vi "laba 9.vi"() -> ()   [LabVIEW 2010]
doc: "Use this template to build a producer/consumer design pattern with events to produce queue items. Use this design pattern instead of the User Interface Event Handler pattern for user interfaces when you want to execute code asynchronously in response to an event without slowing the user interface responsiveness."
uses:
  laba_9_typedef.ctl
panel:
  in  "Start":bool
  out "string":string
  in  "Stop":bool
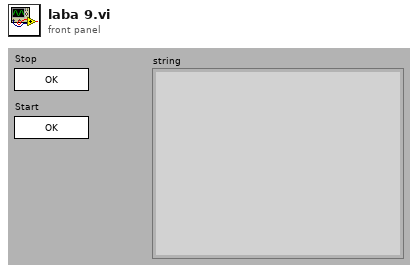
[diagram p1: front panel]
types:
  T1 = typedef "laba_9_typedef.ctl" = enum16{"Initialize", "Read multi", "String view", "Stop"}
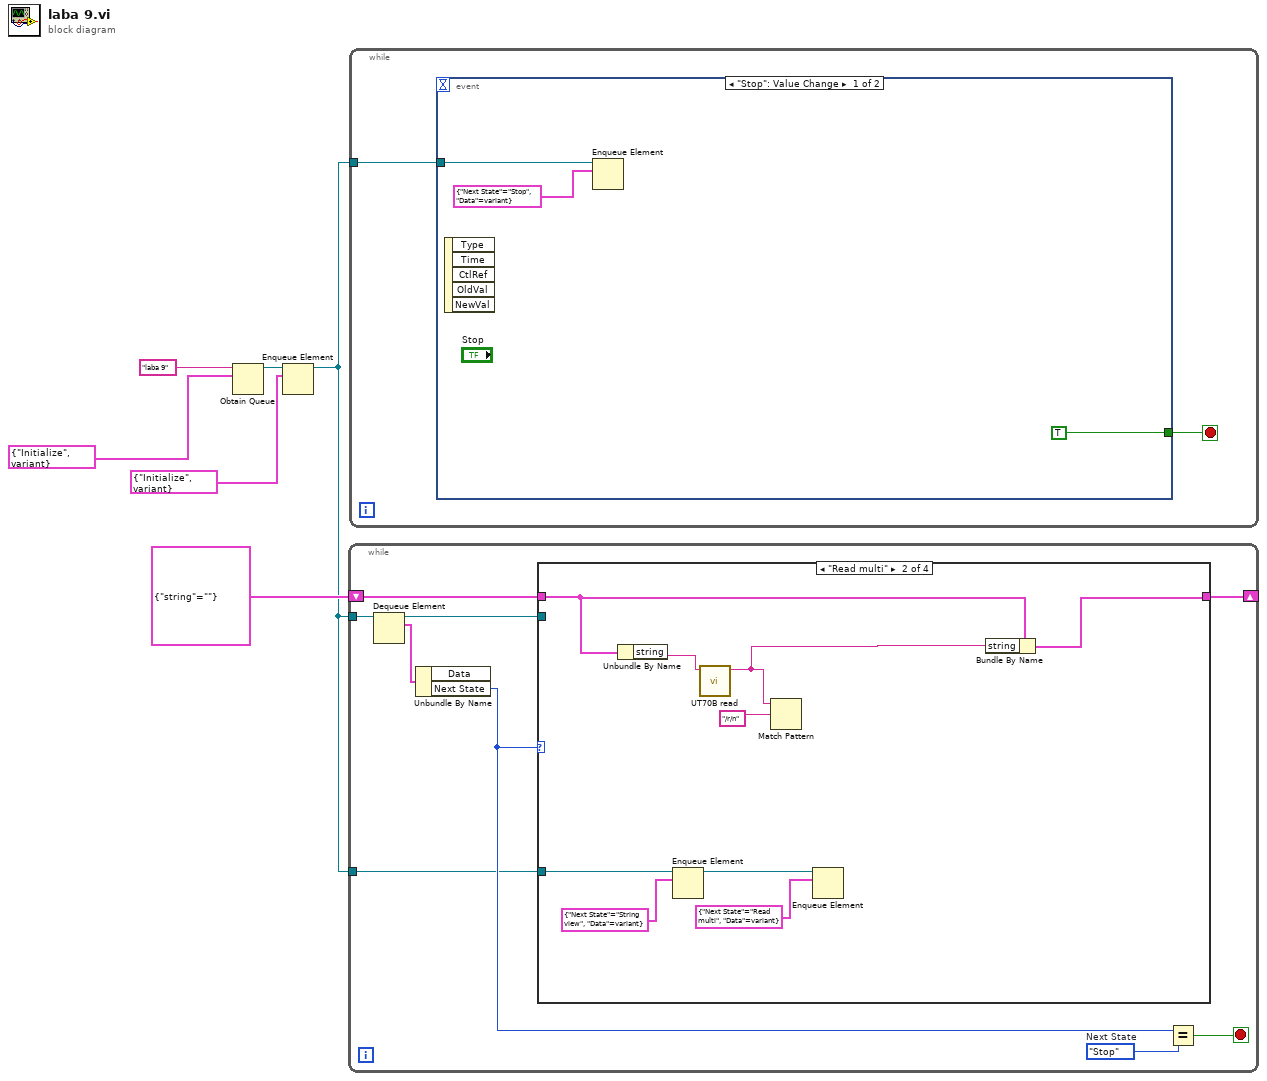
[diagram p0: block diagram]
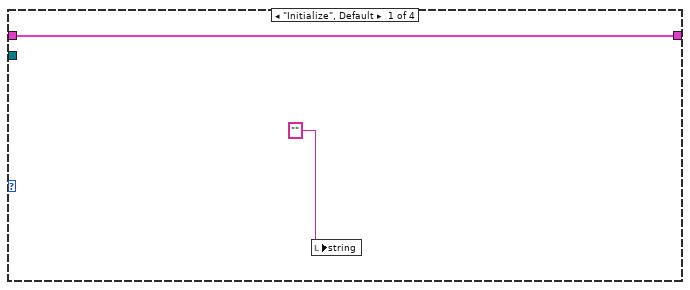
[diagram p2: hidden frame]
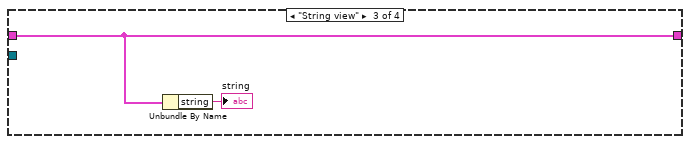
[diagram p3: hidden frame]
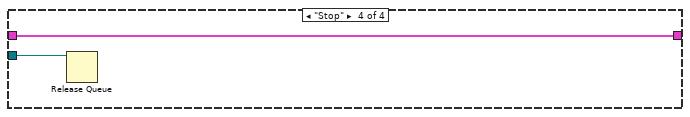
[diagram p4: hidden frame]
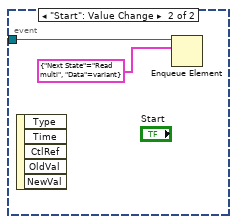
[diagram p5: hidden frame]
diagram:
  n1 = Obtain Queue(name (unnamed)="laba 9", element data type=cluster{"Next State":T1, "Data":variant} {"Next State"=enum."Initialize", "Data"=variant}) -> (queue out=w6:refnum<queue>)  [unwired: 3 in, 2 out]
  n2 = Enqueue Element(queue=w6, element=cluster{"Next State":T1, "Data":variant} {"Next State"=enum."Initialize", "Data"=variant}) -> (queue out=w1:refnum<queue>)  [unwired: 2 in, 2 out]
  n3 = while {
    tunnel: w1 -> [w15]
    shift-right: [w8] -> _
    shift-left: cluster{"string":string} {"string"=""} -> [w9]
    tunnel: w1 -> [w7]
    stop <- w13 stop-if-true
    w12 = laba_9_typedef."Stop"  # Next State
    n4 = Dequeue Element(queue=w15) -> (queue out=w10:refnum<queue>, element=w14:cluster{"Next State":T1, "Data":variant})  [unwired: 2 in, 2 out]
    n5 = Unbundle By Name(w14) -> ("Next State"=w11:T1)  [unwired: 1 out]
    n6 = case shown="\"Read multi\"" w11 {
      tunnel: w10 -> [_ _ _ w30]
      tunnel: w9 -> [w17 w25 w28 w29]
      tunnel: [w17 w24 w28 w29] -> w8
      tunnel: w7 -> [_ w23 _ _]
      frame "Initialize", Default {
        n7 = local write "string"("" ("string")) -> ()
      }
      frame "Read multi" {
        n8 = Unbundle By Name(w25) -> ("string"=w26:string)
        n9 = Enqueue Element(queue=w23, element=cluster{"Next State":T1, "Data":variant} {"Next State"=enum."String view", "Data"=variant}) -> (queue out=w21:refnum<queue>)  [unwired: 2 in, 2 out]
        n10 = call "UT70B read.vi"("string in"=w26) -> ("string out"=w19:string)  [unwired: 10 in]
        n11 = Match Pattern(string=w19, regular expression="/r/n") -> ()  [unwired: 1 in, 4 out]
        n12 = Enqueue Element(queue=w21, element=cluster{"Next State":T1, "Data":variant} {"Next State"=enum."Read multi", "Data"=variant}) -> ()  [unwired: 2 in, 3 out]
        n13 = Bundle By Name(cluster=w25, "string"=w19) -> (w24:cluster{"string":string})
      }
      frame "String view" {
        n14 = Unbundle By Name(w28) -> ("string"=→"string":string)
      }
      frame "Stop" {
        n15 = Release Queue(queue=w30) -> ()  [unwired: 2 in, 3 out]
      }
    }
    n16 = Equal?(x=w11, y=w12) -> (x = y?=w13:bool)
  }
  n17 = while {
    tunnel: w1 -> [w32]
    stop <- w31 stop-if-true
    n18 = event shown="[0] \"Stop\": Value Change" {
      selector: _ -> [_ _]
      dyn-events: _ -> [_ _]
      timeout: _ -> [_ _]
      tunnel: w32 -> [w35 w37]
      tunnel: [TRUE _] -> w31
      event "Stop": Value Change {
        n19 = event-data() -> ()  [unwired: 1 in, 5 out]
        n20 = Enqueue Element(queue=w35, element=cluster{"Next State":T1, "Data":variant} {"Next State"=enum."Stop", "Data"=variant}) -> ()  [unwired: 2 in, 3 out]
      }
      event "Start": Value Change {
        n21 = event-data() -> ()  [unwired: 1 in, 5 out]
        n22 = Enqueue Element(queue=w37, element=cluster{"Next State":T1, "Data":variant} {"Next State"=enum."Read multi", "Data"=variant}) -> ()  [unwired: 2 in, 3 out]
      }
    }
  }
